vi "AD7609 Check overrun.vi"(0 "VISA resource name":refnum<visa-resource-name>) -> (1 "Overruns":u32, 2 "Overrun error out":errorcluster)   [LabVIEW 2020]
uses:
  <vilib>/Instr/_visa.llb/VISA Open Access Mode.ctl
panel:
  out "Overrun string output":string
  # "PN 25/11/2014, 17/08/2015"
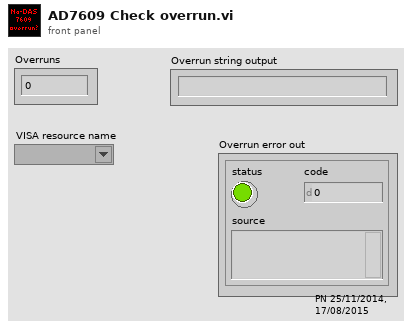
[diagram p1: front panel]
types:
  T1 = typedef "VISA Open Access Mode.ctl" = u32
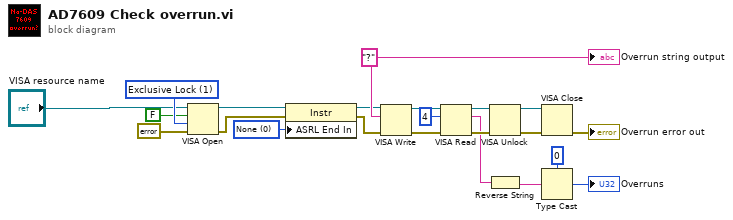
[diagram p0: block diagram]
diagram:
  w6 = u16 0 items=["None", "Last Bit", "TermChar"] ("Serial Settings:End Mode for Reads")
  w22 = T1 1 items=["VISA Defaults"=0, "Exclusive Lock"=1, "Load Configured Settings"=4] ("Access Mode")
  w16 = "?"
  n1 = VISA Open(duplicate session (F)=FALSE, access mode=w22, error in (no error)=errorcluster {"status"=FALSE, "code"=0, "source"=""}, VISA resource name="VISA resource name") -> (VISA resource name=w5:refnum<visa-resource-name>, error out=w2:errorcluster)  [unwired: 1 in]
  n2 = property class="Instr"(reference=w5, error in=w2, "ASRL End In"=w6) -> (reference out=w4:refnum<visa-resource-name>, error out=w3:errorcluster)
  n3 = VISA Write(VISA resource name=w4, write buffer=w16, error in (no error)=w3) -> (VISA resource name out=w12:refnum<visa-resource-name>, error out=w15:errorcluster)  [unwired: 1 out]
  n4 = VISA Read(VISA resource name=w12, byte count=u32 4, error in (no error)=w15) -> (VISA resource name out=w11:refnum<visa-resource-name>, read buffer=w9:string, error out=w14:errorcluster)  [unwired: 1 out]
  n5 = VISA Unlock(8:w14, 11:w11) -> (0:w19:errorcluster, 3:w20:refnum<visa-resource-name>)
  n6 = Reverse String(1:w9) -> (0:w7:string)
  n7 = VISA Close(VISA resource name=w20, error in (no error)=w19) -> (error out=→"Overrun error out":errorcluster)
  n8 = Type Cast(type=u32 0, x=w7) -> (*(type *) &x=→"Overruns":u32)
  "Overrun string output" <- w16
